vi "Read Event Reg.vi"(2 "EnclaveChannel":T1) -> (7 "Event Reg":refnum<event-registration>)   [LabVIEW 2022 SP3, in "Enclave.lvlib"]
doc: "Creates an event registration directly from the Channel Wire to be used with dynamic event terminals on an event structure. The event also includes a <b>Closed</b> value which will be true when no more data will be received."
uses:
  Enclave.lvlib
  Event/Event.lvclass
  Element.ctl
  ))Channel.ctl
  Enclave Event.ctl
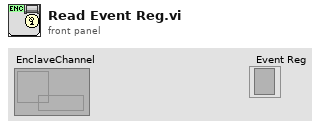
[diagram p1: front panel]
types:
  T1 = typedef "Enclave.lvlib/))Channel.ctl" = refnum<queue>
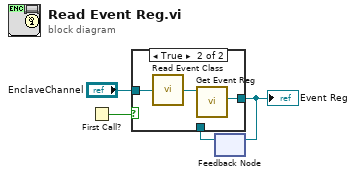
[diagram p0: block diagram]
diagram:
  n1 = First Call?() -> (First Call?: T/F=w4:bool)
  n2 = feedback #1() -> (w1:refnum<event-registration>)  [unwired: 1 in]
  n3 = case shown="True" w4 {
    tunnel: "EnclaveChannel" -> [_ w7]
    tunnel: [w5 w8] -> w2
    tunnel: w1 -> [w5 _]
    frame False {
    }
    frame True {
      n4 = call "Read Event Class.vi"("Enclave"=w7) -> ("Event"=w6:refnum<class "Event.lvclass">)  [unwired: 8 in]
      n5 = call "Get Event Reg.vi"("Event in"=w6) -> ("Event Reg"=w8:refnum<event-registration>)  [unwired: 9 in, 1 out]
    }
  }
  "Event Reg" <- w2
  n6 = feedback-in #1(w2) -> ()
